vi "log analysis_gps.vi"() -> ()   [LabVIEW 2018] (continued)
2 28.000000 0 0\trobot status\t224.451032\t106.284325\t8.226800\t-0.416933\t-0.582279\t162.075425\t0.000000\t0.000000\n\t\n15:38:05.2\tlog_raw\tgps_raw\t\tsystem status\tnormal 2 28.000000 0 0\trobot status\t224.451188\t106.284516\t8.226800\t-0.415432\t-0.584104\t162.073380\t0.000000\t0.000000\n\t\n15:38:05.7\tlog_raw\tgps_raw\t#INSPVAXA,USB3,0,48.5,FINESTEERING,2107,283103.750,02000000,471d,15824;INS_ALIGNMENT_COMPLETE,INS_RTKFIXED,37.37108788000,126.72336903510,8.2270,22.3000,0.0050,0.0045,0.0003,-0.414277574,-0.583463216,287.925982879,0.2110,0.1573,0.2695,0.0344,0.0343,0.0312,0.0795,0.0805,4.9172,0f000005,0*7ee9c1ee\n\tsystem status\tnormal 2 28.000000 0 0\trobot status\t224.451369\t106.285108\t8.227000\t-0.414278\t-0.583463\t162.074017\t0.000000\t0.000000\n\t\n15:38:06.2\tlog_raw\tgps_raw\t#INSPVAXA,USB3,0,49.0,FINESTEERING,2107,283104.250,02000000,471d,15824;INS_ALIGNMENT_COMPLETE,INS_RTKFIXED,37.37108788419,126.72336903801,8.2270,22.3000,0.0052,0.0047,-0.0002,-0.414476277,-0.584193509,287.926239450,0.2108,0.1573,0.2688,0.0344,0.0343,0.0312,0.0795,0.0805,4.9186,0f000005,0*7089b505\n\tsystem status\tnormal 2 28.000000 0 0\trobot status\t224.451627\t106.285573\t8.227000\t-0.414476\t-0.584194\t162.073761\t0.000000\t0.000000\n\t\n15:38:06.7\tlog_raw\tgps_raw\t#INSPVAXA,USB3,0,49.0,FINESTEERING,2107,283104.750,02000000,471d,15824;INS_ALIGNMENT_COMPLETE,INS_RTKFIXED,37.37108788145,126.72336903923,8.2266,22.3000,0.0045,0.0040,-0.0007,-0.415917885,-0.588202727,287.926434552,0.2108,0.1573,0.2688,0.0344,0.0343,0.0312,0.0795,0.0805,4.9186,0f000005,0*a8fd5de4\n\tsystem status\tnormal 2 28.000000 0 0\trobot status\t224.451735\t106.285269\t8.226600\t-0.415918\t-0.588203\t162.073565\t0.000000\t0.000000\n\t\n15:38:07.2\tlog_raw\tgps_raw\t#INSPVAXA,USB3,0,48.0,FINESTEERING,2107,283105.250,02000000,471d,15824;INS_ALIGNMENT_COMPLETE,INS_RTKFIXED,37.37108788026,126.72336903795,8.2263,22.3000,0.0046,0.0032,-0.0010,-0.414361935,-0.591993164,287.925953212,0.2107,0.1573,0.2682,0.0344,0.0343,0.0312,0.0795,0.0805,4.9201,0f000005,0*118aea77\n\tsystem status\tnormal 2 28.000000 0 0\trobot status\t224.451622\t106.285136\t8.226300\t-0.414362\t-0.591993\t162.074047\t0.000000\t0.000000\n\t\n15:38:07.7\tlog_raw\tgps_raw\t#INSPVAXA,USB3,0,48.0,FINESTEERING,2107,283105.750,02000000,471d,15824;INS_ALIGNMENT_COMPLETE,INS_RTKFIXED,37.37108788332,126.72336903309,8.2260,22.3000,0.0050,0.0029,-0.0017,-0.412327684,-0.591969420,287.923357283,0.2107,0.1573,0.2682,0.0344,0.0343,0.0312,0.0795,0.0805,4.9201,0f000005,0*6e4f183a\n\tsystem status\tnormal 2 28.000000 0 0\trobot status\t224.451191\t106.285476\t8.226000\t-0.412328\t-0.591969\t162.076643\t0.000000\t0.000000\n\t\n15:38:08.2\tlog_raw\tgps_raw\t#INSPVAXA,USB3,0,48.5,FINESTEERING,2107,283106.250,02000000,471d,15824;INS_ALIGNMENT_COMPLETE,INS_RTKFIXED,37.37108788583,126.72336903030,8.2257,22.3000,0.0061,0.0025,-0.0021,-0.413322314,-0.593362730,287.923193741,0.2106,0.1573,0.2676,0.0344,0.0343,0.0312,0.0795,0.0805,4.9216,0f000005,0*8b1995f2\n\tsystem status\tnormal 2 28.000000 0 0\trobot status\t224.450944\t106.285755\t8.225700\t-0.413322\t-0.593363\t162.076806\t0.000000\t0.000000\n\t\n15:38:08.7\tlog_raw\tgps_raw\t#INSPVAXA,USB3,0,48.5,FINESTEERING,2107,283106.750,02000000,471d,15824;INS_ALIGNMENT_COMPLETE,INS_RTKFIXED,37.37108788780,126.72336903040,8.2256,22.3000,0.0063,0.0024,-0.0014,-0.411919741,-0.593309816,287.922053260,0.2106,0.1573,0.2676,0.0344,0.0343,0.0312,0.0795,0.0805,4.9216,0f000005,0*86796b00\n\tsystem status\tnormal 2 28.000000 0 0\trobot status\t224.450953\t106.285973\t8.225600\t-0.411920\t-0.593310\t162.077947\t0.000000\t0.000000\n\t\n15:38:09.2\tlog_raw\tgps_raw\t\tsystem status\tnormal 2 28.000000 0 0\trobot status\t224.450894\t106.286027\t8.225400\t-0.411158\t-0.594185\t162.080368\t0.000000\t0.000000\n\t\n15:38:09.7\tlog_raw\tgps_raw\t\tsystem status\tnormal 2 28.000000 0 0\trobot status\t224.450634\t106.285755\t8.225200\t-0.409687\t-0.594930\t162.079773\t0.000000\t0.000000\n\t\n15:38:10.2\tlog_raw\tgps_raw\t#INSPVAXA,USB3,0,49.0,FINESTEERING,2107,283108.250,02000000,471d,15824;INS_ALIGNMENT_COMPLETE,INS_RTKFIXED,37.37108788248,126.72336902361,8.2250,22.3000,0.0042,0.0015,-0.0018,-0.409863659,-0.598671820,287.918736221,0.2106,0.1573,0.2666,0.0344,0.0343,0.0312,0.0795,0.0805,4.9245,0f000005,0*9ed896c6\n\tsystem status\tnormal 2 28.000000 0 0\trobot status\t224.450352\t106.285383\t8.225000\t-0.409864\t-0.598672\t162.081264\t0.000000\t0.000000\n\t\n15:38:10.7\tlog_raw\tgps_raw\t#INSPVAXA,USB3,0,49.0,FINESTEERING,2107,283108.750,02000000,471d,15824;INS_ALIGNMENT_COMPLETE,INS_RTKFIXED,37.37108788055,126.72336902250,8.2249,22.3000,0.0042,0.0020,-0.0022,-0.409039214,-0.598045025,287.918760673,0.2106,0.1573,0.2666,0.0344,0.0343,0.0312,0.0795,0.0805,4.9245,0f000005,0*7d4209e8\n\tsystem status\tnormal 2 28.000000 0 0\trobot status\t224.450253\t106.285169\t8.224900\t-0.409039\t-0.598045\t162.081239\t0.000000\t0.000000\n\t\n15:38:11.2\tlog_raw\tgps_raw\t#INSPVAXA,USB3,0,49.0,FINESTEERING,2107,283109.250,02000000,471d,15824;INS_ALIGNMENT_COMPLETE,INS_RTKFIXED,37.37108788018,126.72336902226,8.2247,22.3000,0.0041,0.0020,-0.0021,-0.409961189,-0.600264889,287.916717631,0.2105,0.1573,0.2661,0.0344,0.0343,0.0312,0.0795,0.0805,4.9260,0f000005,0*bcf00a2d\n\tsystem status\tnormal 2 28.000000 0 0\trobot status\t224.450232\t106.285128\t8.224700\t-0.409961\t-0.600265\t162.083282\t0.000000\t0.000000\n\t\n15:38:11.7\tlog_raw\tgps_raw\t#INSPVAXA,USB3,0,49.0,FINESTEERING,2107,283109.750,02000000,471d,15824;INS_ALIGNMENT_COMPLETE,INS_RTKFIXED,37.37108788128,126.72336902017,8.2243,22.3000,0.0038,0.0017,-0.0025,-0.411876741,-0.602713375,287.916096171,0.2105,0.1573,0.2661,0.0344,0.0343,0.0312,0.0795,0.0805,4.9260,0f000005,0*0e51d129\n\tsystem status\tnormal 2 28.000000 0 0\trobot status\t224.450047\t106.285250\t8.224300\t-0.411877\t-0.602713\t162.083904\t0.000000\t0.000000\n\t\n15:38:12.2\tlog_raw\tgps_raw\t#INSPVAXA,USB3,0,47.0,FINESTEERING,2107,283110.250,02000000,471d,15824;INS_ALIGNMENT_COMPLETE,INS_RTKFIXED,37.37108788100,126.72336901819,8.2239,22.3000,0.0037,0.0018,-0.0030,-0.411621660,-0.604000034,287.914564647,0.2104,0.1573,0.2657,0.0344,0.0343,0.0312,0.0795,0.0805,4.9275,0f000005,0*d6cead36\n\tsystem status\tnormal 2 28.000000 0 0\trobot status\t224.449871\t106.285219\t8.223900\t-0.411622\t-0.604000\t162.085435\t0.000000\t0.000000\n\t\n15:38:12.7\tlog_raw\tgps_raw\t#INSPVAXA,USB3,0,47.0,FINESTEERING,2107,283110.750,02000000,471d,15824;INS_ALIGNMENT_COMPLETE,INS_RTKFIXED,37.37108787882,126.72336901490,8.2238,22.3000,0.0031,0.0013,-0.0034,-0.411270923,-0.605029312,287.914838543,0.2104,0.1573,0.2657,0.0344,0.0343,0.0312,0.0795,0.0805,4.9275,0f000005,0*6d07f4f4\n\tsystem status\tnormal 2 28.000000 0 0\trobot status\t224.449580\t106.284977\t8.223800\t-0.411271\t-0.605029\t162.085161\t0.000000\t0.000000\n\t\n15:38:13.2\tlog_raw\tgps_raw\t#INSPVAXA,USB3,0,44.0,FINESTEERING,2107,283111.250,02000000,471d,15824;INS_ALIGNMENT_COMPLETE,INS_RTKFIXED,37.37108787798,126.72336901339,8.2237,22.3000,0.0035,0.0008,-0.0027,-0.411014484,-0.606801614,287.916144015,0.2104,0.1572,0.2653,0.0344,0.0343,0.0312,0.0795,0.0805,4.9290,0f000005,0*17fda63e\n\tsystem status\tnormal 2 28.000000 0 0\trobot status\t224.449446\t106.284883\t8.223700\t-0.411014\t-0.606802\t162.083856\t0.000000\t0.000000\n\t\n15:38:13.7\tlog_raw\tgps_raw\t\tsystem status\tnormal 2 28.000000 0 0\trobot status\t224.449134\t106.285474\t8.223900\t-0.409737\t-0.609292\t162.084146\t0.000000\t0.000000\n\t\n15:38:14.2\tlog_raw\tgps_raw\t#INSPVAXA,USB3,0,46.5,FINESTEERING,2107,283112.250,02000000,471d,15824;INS_ALIGNMENT_COMPLETE,INS_RTKFIXED,37.37108788668,126.72336900523,8.2241,22.3000,0.0049,-0.0005,-0.0016,-0.408777501,-0.612185293,287.914677114,0.2103,0.1572,0.2649,0.0344,0.0343,0.0312,0.0795,0.0805,4.9305,0f000005,0*82ade194\n\tsystem status\tnormal 2 28.000000 0 0\trobot status\t224.448723\t106.285849\t8.224100\t-0.408778\t-0.612185\t162.085323\t0.000000\t0.000000\n\t\n15:38:14.7\tlog_raw\tgps_raw\t#INSPVAXA,USB3,0,46.5,FINESTEERING,2107,283112.750,02000000,471d,15824;INS_ALIGNMENT_COMPLETE,INS_RTKFIXED,37.37108788778,126.72336899951,8.2242,22.3000,0.0047,-0.0009,-0.0019,-0.409122282,-0.611972311,287.914890224,0.2103,0.1572,0.2649,0.0344,0.0343,0.0312,0.0795,0.0805,4.9305,0f000005,0*c3a4b162\n\tsystem status\tnormal 2 28.000000 0 0\trobot status\t224.448217\t106.285971\t8.224200\t-0.409122\t-0.611972\t162.085110\t0.000000\t0.000000\n\t\n15:38:15.2\tlog_raw\tgps_raw\t#INSPVAXA,USB3,0,48.5,FINESTEERING,2107,283113.250,02000000,471d,15824;INS_ALIGNMENT_COMPLETE,INS_RTKFIXED,37.37108788861,126.72336899425,8.2243,22.3000,0.0050,-0.0013,-0.0019,-0.410508140,-0.611024198,287.914176571,0.2103,0.1572,0.2646,0.0344,0.0343,0.0312,0.0795,0.0805,4.9321,0f000005,0*87d2d5b6\n\tsystem status\tnormal 2 28.000000 0 0\trobot status\t224.447751\t106.286063\t8.224300\t-0.410508\t-0.611024\t162.085823\t0.000000\t0.000000\n\t\n15:38:15.7\tlog_raw\tgps_raw\t#INSPVAXA,USB3,0,48.5,FINESTEERING,2107,283113.750,02000000,471d,15824;INS_ALIGNMENT_COMPLETE,INS_RTKFIXED,37.37108789363,126.72336898840,8.2244,22.3000,0.0063,-0.0021,-0.0017,-0.411022705,-0.609051513,287.913579305,0.2103,0.1572,0.2646,0.0344,0.0343,0.0312,0.0795,0.0805,4.9321,0f000005,0*35e79e67\n\tsystem status\tnormal 2 28.000000 0 0\trobot status\t224.447233\t106.286620\t8.224400\t-0.411023\t-0.609052\t162.086421\t0.000000\t0.000000\n\t\n15:38:16.2\tlog_raw\tgps_raw\t#INSPVAXA,USB3,0,47.0,FINESTEERING,2107,283114.250,02000000,471d,15824;INS_ALIGNMENT_COMPLETE,INS_RTKFIXED,37.37108789523,126.72336898295,8.2245,22.3000,0.0061,-0.0024,-0.0023,-0.410389175,-0.608679796,287.908436695,0.2102,0.1572,0.2643,0.0344,0.0343,0.0312,0.0795,0.0805,4.9336,0f000005,0*e900128e\n\tsystem status\tnormal 2 28.000000 0 0\trobot status\t224.446750\t106.286798\t8.224500\t-0.410389\t-0.608680\t162.091563\t0.000000\t0.000000\n\t\n15:38:16.7\tlog_raw\tgps_raw\t#INSPVAXA,USB3,0,47.0,FINESTEERING,2107,283114.750,02000000,471d,15824;INS_ALIGNMENT_COMPLETE,INS_RTKFIXED,37.37108789043,126.72336897889,8.2245,22.3000,0.0054,-0.0027,-0.0027,-0.410079836,-0.608000188,287.907030910,0.2102,0.1572,0.2643,0.0344,0.0343,0.0312,0.0795,0.0805,4.9336,0f000005,0*f5aa2bf4\n\tsystem status\tnormal 2 28.000000 0 0\trobot status\t224.446390\t106.286265\t8.224500\t-0.410080\t-0.608000\t162.092969\t0.000000\t0.000000\n\t\n15:38:17.2\tlog_raw\tgps_raw\t#INSPVAXA,USB3,0,46.0,FINESTEERING,2107,283115.250,02000000,471d,15824;INS_ALIGNMENT_COMPLETE,INS_RTKFIXED,37.37108788786,126.72336897498,8.2245,22.3000,0.0055,-0.0029,-0.0021,-0.409736809,-0.602715261,287.905938302,0.2101,0.1572,0.2640,0.0344,0.0343,0.0312,0.0795,0.0805,4.9352,0f000005,0*b8856e6c\n\tsystem status\tnormal 2 28.000000 0 0\trobot status\t224.446044\t106.285980\t8.224500\t-0.409737\t-0.602715\t162.094062\t0.000000\t0.000000\n\t\n15:38:17.7\tlog_raw\tgps_raw\t#INSPVAXA,USB3,0,46.0,FINESTEERING,2107,283115.750,02000000,471d,15824;INS_ALIGNMENT_COMPLETE,INS_RTKFIXED,37.37108788493,126.72336897577,8.2245,22.3000,0.0046,-0.0023,-0.0026,-0.410098984,-0.602405796,287.902959038,0.2101,0.1572,0.2640,0.0344,0.0343,0.0312,0.0795,0.0805,4.9352,0f000005,0*5724c76a\n\tsystem status\tnormal 2 28.000000 0 0\trobot status\t224.446114\t106.285655\t8.224500\t-0.410099\t-0.602406\t162.097041\t0.000000\t0.000000\n\t\n15:38:18.2\tlog_raw\tgps_raw\t\tsystem status\tnormal 2 28.000000 0 0\trobot status\t224.446206\t106.285296\t8.224400\t-0.410302\t-0.600878\t162.097351\t0.000000\t0.000000\n\t\n15:38:18.7\tlog_raw\tgps_raw\t\tsystem status\tnormal 2 28.000000 0 0\trobot status\t224.446412\t106.285047\t8.224500\t-0.408719\t-0.597692\t162.099652\t0.000000\t0.000000\n\t\n15:38:19.2\tlog_raw\tgps_raw\t#INSPVAXA,USB3,0,48.5,FINESTEERING,2107,283117.250,02000000,471d,15824;INS_ALIGNMENT_COMPLETE,INS_RTKFIXED,37.37108787822,126.72336898248,8.2247,22.3000,0.0046,0.0006,-0.0022,-0.408932053,-0.597708499,287.898385765,0.2100,0.1572,0.2634,0.0344,0.0343,0.0312,0.0795,0.0805,4.9381,0f000005,0*450763d8\n\tsystem status\tnormal 2 28.000000 0 0\trobot status\t224.446708\t106.284910\t8.224700\t-0.408932\t-0.597708\t162.101614\t0.000000\t0.000000\n\t\n15:38:19.7\tlog_raw\tgps_raw\t\tsystem status\tnormal 2 28.000000 0 0\trobot status\t224.446942\t106.284576\t8.225000\t-0.409149\t-0.598860\t162.102968\t0.000000\t0.000000\n\t\n15:38:20.2\tlog_raw\tgps_raw\t\tsystem status\tnormal 2 28.000000 0 0\trobot status\t224.447153\t106.284340\t8.225300\t-0.409921\t-0.598794\t162.103793\t0.000000\t0.000000\n\t\n15:38:20.7\tlog_raw\tgps_raw\t#INSPVAXA,USB3,0,51.5,FINESTEERING,2107,283118.750,02000000,471d,15824;INS_ALIGNMENT_COMPLETE,INS_RTKFIXED,37.37108787489,126.72336898888,8.2255,22.3000,0.0051,0.0006,-0.0004,-0.410553255,-0.597325999,287.895855349,0.2099,0.1572,0.2632,0.0344,0.0343,0.0312,0.0794,0.0805,4.9396,0f000005,0*531bbf8e\n\tsystem status\tnormal 2 28.000000 0 0\trobot status\t224.447275\t106.284541\t8.225500\t-0.410553\t-0.597326\t162.104145\t0.000000\t0.000000\n\t\n15:38:21.2\tlog_raw\tgps_raw\t\tsystem status\tnormal 2 28.000000 0 0\trobot status\t224.447208\t106.284839\t8.225600\t-0.411045\t-0.597182\t162.104666\t0.000000\t0.000000\n\t\n15:38:21.7\tlog_raw\tgps_raw\t#INSPVAXA,USB3,0,49.0,FINESTEERING,2107,283119.750,02000000,471d,15824;INS_ALIGNMENT_COMPLETE,INS_RTKFIXED,37.37108788239,126.72336898736,8.2256,22.3000,0.0062,0.0005,-0.0005,-0.410245690,-0.596223685,287.896349306,0.2099,0.1572,0.2630,0.0344,0.0343,0.0312,0.0794,0.0805,4.9410,0f000005,0*aabca186\n\tsystem status\tnormal 2 28.000000 0 0\trobot status\t224.447141\t106.285373\t8.225600\t-0.410246\t-0.596224\t162.103651\t0.000000\t0.000000\n\t\n15:38:22.2\tlog_raw\tgps_raw\t#INSPVAXA,USB3,0,47.5,FINESTEERING,2107,283120.250,02000000,471d,15824;INS_ALIGNMENT_COMPLETE,INS_RTKFIXED,37.37108788462,126.72336898711,8.2255,22.3000,0.0062,0.0002,-0.0014,-0.410019875,-0.596819628,287.894466218,0.2099,0.1572,0.2628,0.0344,0.0343,0.0312,0.0794,0.0805,4.9425,0f000005,0*feb71611\n\tsystem status\tnormal 2 28.000000 0 0\trobot status\t224.447118\t106.285620\t8.225500\t-0.410020\t-0.596820\t162.105534\t0.000000\t0.000000\n\t\n15:38:22.7\tlog_raw\tgps_raw\t\tsystem status\tnormal 2 28.000000 0 0\trobot status\t224.447175\t106.285403\t8.225200\t-0.411640\t-0.595952\t162.105189\t0.000000\t0.000000\n\t\n15:38:23.2\tlog_raw\tgps_raw\t#INSPVAXA,USB3,0,47.5,FINESTEERING,2107,283121.250,02000000,471d,15824;INS_ALIGNMENT_COMPLETE,INS_RTKFIXED,37.37108788020,126.72336899019,8.2251,22.3000,0.0049,0.0012,-0.0017,-0.410504520,-0.596359600,287.895045223,0.2098,0.1572,0.2627,0.0344,0.0343,0.0312,0.0794,0.0805,4.9439,0f000005,0*861abdab\n\tsystem status\tnormal 2 28.000000 0 0\trobot status\t224.447391\t106.285130\t8.225100\t-0.410505\t-0.596360\t162.104955\t0.000000\t0.000000\n\t\n15:38:23.7\tlog_raw\tgps_raw\t\tsystem status\tnormal 2 28.000000 0 0\trobot status\t224.447275\t106.285221\t8.225400\t-0.410985\t-0.596680\t162.105710\t0.000000\t0.000000\n\t\n15:38:24.2\tlog_raw\tgps_raw\t#INSPVAXA,USB3,0,48.0,FINESTEERING,2107,283122.250,02000000,471d,15824;INS_ALIGNMENT_COMPLETE,INS_RTKFIXED,37.37108788140,126.72336898679,8.2256,22.3000,0.0046,0.0003,-0.0020,-0.412214067,-0.597500472,287.894257245,0.2098,0.1572,0.2625,0.0344,0.0343,0.0312,0.0794,0.0805,4.9454,0f000005,0*41de74d7\n\tsystem status\tnormal 2 28.000000 0 0\trobot status\t224.447090\t106.285263\t8.225600\t-0.412214\t-0.597500\t162.105743\t0.000000\t0.000000\n\t\n15:38:24.7\tlog_raw\tgps_raw\t\tsystem status\tnormal 2 28.000000 0 0\trobot status\t224.447403\t106.284767\t8.225500\t-0.410260\t-0.595330\t162.106312\t0.000000\t0.000000\n\t\n15:38:25.2\tlog_raw\tgps_raw\t\tsystem status\tnormal 2 28.000000 0 0\trobot status\t224.447705\t106.284349\t8.225700\t-0.410048\t-0.596707\t162.108461\t0.000000\t0.000000\n\t\n15:38:25.7\tlog_raw\tgps_raw\t\tsystem status\tnormal 2 28.000000 0 0\trobot status\t224.447585\t106.284234\t8.226100\t-0.411201\t-0.596838\t162.109642\t0.000000\t0.000000\n\t\n15:38:26.2\tlog_raw\tgps_raw\t\tsystem status\tnormal 2 28.000000 0 0\trobot status\t224.447570\t106.283848\t8.226500\t-0.410870\t-0.598506\t162.111627\t0.000000\t0.000000\n\t\n15:38:26.7\tlog_raw\tgps_raw\t\tsystem status\tnormal 2 28.000000 0 0\trobot status\t224.447639\t106.283383\t8.226500\t-0.408777\t-0.600718\t162.112837\t0.000000\t0.000000\n\t\n15:38:27.2\tlog_raw\tgps_raw\t\tsystem status\tnormal 2 28.000000 0 0\trobot status\t224.447605\t106.283011\t8.226500\t-0.406755\t-0.601265\t162.115733\t0.000000\t0.000000\n\t\n15:38:27.7\tlog_raw\tgps_raw\t\tsystem status\tnormal 2 28.000000 0 0\trobot status\t224.447669\t106.282715\t8.226400\t-0.405589\t-0.600901\t162.115380\t0.000000\t0.000000\n\t\n15:38:28.2\tlog_raw\tgps_raw\t#INSPVAXA,USB3,0,46.5,FINESTEERING,2107,283126.250,02000000,471d,15824;INS_ALIGNMENT_COMPLETE,INS_RTKFIXED,37.37108785781,126.72336899407,8.2263,22.3000,0.0034,0.0010,-0.0014,-0.405163325,-0.599911050,287.885200973,0.2098,0.1572,0.2620,0.0344,0.0343,0.0312,0.0794,0.0804,4.9511,0f000005,0*554930fc\n\tsystem status\tnormal 2 28.000000 0 0\trobot status\t224.447735\t106.282645\t8.226300\t-0.405163\t-0.599911\t162.114799\t0.000000\t0.000000\n\t\n15:38:28.7\tlog_raw\tgps_raw\t\tsystem status\tnormal 2 28.000000 0 0\trobot status\t224.447887\t106.282579\t8.226100\t-0.406198\t-0.601239\t162.115348\t0.000000\t0.000000\n\t\n15:38:29.2\tlog_raw\tgps_raw\t\tsystem status\tnormal 2 28.000000 0 0\trobot status\t224.447997\t106.282609\t8.225900\t-0.407404\t-0.600387\t162.116168\t0.000000\t0.000000\n\t\n15:38:29.7\tlog_raw\tgps_raw\t\tsystem status\tnormal 2 28.000000 0 0\trobot status\t224.448154\t106.282775\t8.225900\t-0.406329\t-0.599457\t162.114574\t0.000000\t0.000000\n\t\n15:38:30.2\tlog_raw\tgps_raw\t\tsystem status\tnormal 2 28.000000 0 0\trobot status\t224.448312\t106.282869\t8.225900\t-0.405480\t-0.599703\t162.115826\t0.000000\t0.000000\n\t\n15:38:30.7\tlog_raw\tgps_raw\t\tsystem status\tnormal 2 28.000000 0 0\trobot status\t224.448419\t106.282962\t8.225800\t-0.403880\t-0.599318\t162.116186\t0.000000\t0.000000\n\t\n15:38:31.2\tlog_raw\tgps_raw\t\tsystem status\tnormal 2 28.000000 0 0\trobot status\t224.448426\t106.283107\t8.225500\t-0.401514\t-0.597654\t162.115583\t0.000000\t0.000000\n\t\n15:38:31.7\tlog_raw\tgps_raw\t\tsystem status\tnormal 2 28.000000 0 0\trobot status\t224.448410\t106.283254\t8.225400\t-0.401145\t-0.595126\t162.115399\t0.000000\t0.000000\n\t\n15:38:32.2\tlog_raw\tgps_raw\t\tsystem status\tnormal 2 28.000000 0 0\trobot status\t224.448462\t106.283450\t8.225300\t-0.398774\t-0.594293\t162.114275\t0.000000\t0.000000\n\t\n15:38:32.7\tlog_raw\tgps_raw\t\tsystem status\tnormal 2 28.000000 0 0\trobot status\t224.448562\t106.283708\t8.225500\t-0.399325\t-0.595095\t162.114742\t0.000000\t0.000000\n\t\n15:38:33.2\tlog_raw\tgps_raw\t\tsystem status\tnormal 2 28.000000 0 0\trobot status\t224.448698\t106.283907\t8.225600\t-0.399060\t-0.595550\t162.114322\t0.000000\t0.000000\n\t\n15:38:33.7\tlog_raw\tgps_raw\t\tsystem status\tnormal 2 28.000000 0 0\trobot status\t224.449149\t106.284287\t8.225700\t-0.398384\t-0.595717\t162.114541\t0.000000\t0.000000\n\t\n15:38:34.2\tlog_raw\tgps_raw\t\tsystem status\tnormal 2 28.000000 0 0\trobot status\t224.449553\t106.284564\t8.225700\t-0.399591\t-0.594833\t162.114493\t0.000000\t0.000000\n\t\n15:38:34.7\tlog_raw\tgps_raw\t\tsystem status\tnormal 2 28.000000 0 0\trobot status\t224.449775\t106.284492\t8.225300\t-0.400663\t-0.594497\t162.113796\t0.000000\t0.000000\n\t\n15:38:35.2\tlog_raw\tgps_raw\t#INSPVAXA,USB3,0,50.5,FINESTEERING,2107,283133.250,02008000,471d,15824;INS_ALIGNMENT_COMPLETE,INS_RTKFIXED,37.37108787441,126.72336901696,8.2251,22.3000,0.0051,0.0025,0.0013,-0.401038405,-0.592309574,287.886306258,0.2098,0.1572,0.2615,0.0344,0.0343,0.0312,0.0794,0.0804,4.9611,0f000005,0*3f736d45\n\tsystem status\tnormal 2 28.000000 0 0\trobot status\t224.449763\t106.284487\t8.225100\t-0.401038\t-0.592310\t162.113694\t0.000000\t0.000000\n\t\n15:38:35.7\tlog_raw\tgps_raw\t\tsystem status\tnormal 2 28.000000 0 0\trobot status\t224.449857\t106.284844\t8.225400\t-0.401355\t-0.592289\t162.114419\t0.000000\t0.000000\n\t\n15:38:36.2\tlog_raw\tgps_raw\t\tsystem status\tnormal 2 28.000000 0 0\trobot status\t224.450031\t106.285085\t8.225500\t-0.401303\t-0.591132\t162.115391\t0.000000\t0.000000\n\t\n15:38:36.7\tlog_raw\tgps_raw\t\tsystem status\tnormal 2 28.000000 0 0\trobot status\t224.450093\t106.285122\t8.225700\t-0.403482\t-0.591750\t162.114729\t0.000000\t0.000000\n\t\n15:38:37.2\tlog_raw\tgps_raw\t\tsystem status\tnormal 2 28.000000 0 0\trobot status\t224.450414\t106.285141\t8.225700\t-0.404978\t-0.591486\t162.114393\t0.000000\t0.000000\n\t\n15:38:37.7\tlog_raw\tgps_raw\t\tsystem status\tnormal 2 28.000000 0 0\trobot status\t224.451129\t106.285112\t8.225400\t-0.405382\t-0.592732\t162.113860\t0.000000\t0.000000\n\t\n15:38:38.2\tlog_raw\tgps_raw\t\tsystem status\tnormal 2 28.000000 0 0\trobot status\t224.451492\t106.285138\t8.225200\t-0.406408\t-0.593386\t162.114550\t0.000000\t0.000000\n\t\n15:38:38.7\tlog_raw\tgps_raw\t\tsystem status\tnormal 2 28.000000 0 0\trobot status\t224.451405\t106.285118\t8.224900\t-0.407947\t-0.592162\t162.114919\t0.000000\t0.000000\n\t\n15:38:39.2\tlog_raw\tgps_raw\t\tsystem status\tnormal 2 28.000000 0 0\trobot status\t224.451215\t106.285206\t8.224600\t-0.409714\t-0.592940\t162.113033\t0.000000\t0.000000\n\t\n15:38:39.7\tlog_raw\tgps_raw\t\tsystem status\tnormal 2 28.000000 0 0\trobot status\t224.451197\t106.285185\t8.224200\t-0.410417\t-0.593710\t162.112017\t0.000000\t0.000000\n\t\n15:38:40.2\tlog_raw\tgps_raw\t\tsystem status\tnormal 2 28.000000 0 0\trobot status\t224.451087\t106.285125\t8.223800\t-0.410324\t-0.597206\t162.111988\t0.000000\t0.000000\n\t\n15:38:40.7\tlog_raw\tgps_raw\t\tsystem status\tnormal 2 28.000000 0 0\trobot status\t224.450903\t106.285100\t8.223300\t-0.410450\t-0.598032\t162.111967\t0.000000\t0.000000\n\t\n15:38:41.3\tlog_raw\tgps_raw\t\tsystem status\tnormal 2 28.000000 0 0\trobot status\t224.450585\t106.285039\t8.222700\t-0.408179\t-0.598817\t162.113262\t0.000000\t0.000000\n\t\n15:38:41.8\tlog_raw\tgps_raw\t\tsystem status\tnormal 2 28.000000 0 0\trobot status\t224.449934\t106.285203\t8.222300\t-0.409129\t-0.601002\t162.114314\t0.000000\t0.000000\n\t\n15:38:42.3\tlog_raw\tgps_raw\t\tsystem status\tnormal 2 28.000000 0 0\trobot status\t224.449799\t106.285271\t8.222000\t-0.410425\t-0.600335\t162.112811\t0.000000\t0.000000\n\t\n15:38:42.8\tlog_raw\tgps_raw\t\tsystem status\tnormal 2 28.000000 0 0\trobot status\t224.450317\t106.284770\t8.221800\t-0.411049\t-0.600342\t162.114798\t0.000000\t0.000000\n\t\n15:38:43.3\tlog_raw\tgps_raw\t\tsystem status\tnormal 2 28.000000 0 0\trobot status\t224.450564\t106.284254\t8.221600\t-0.410176\t-0.599924\t162.113590\t0.000000\t0.000000\n\t\n15:38:43.8\tlog_raw\tgps_raw\t\tsystem status\tnormal 2 28.000000 0 0\trobot status\t224.450436\t106.283367\t8.221300\t-0.411311\t-0.599715\t162.114209\t0.000000\t0.000000\n\t\n15:38:44.3\tlog_raw\tgps_raw\t\tsystem status\tnormal 2 28.000000 0 0\trobot status\t224.450212\t106.282766\t8.221200\t-0.411664\t-0.598224\t162.112656\t0.000000\t0.000000\n\t\n15:38:44.8\tlog_raw\tgps_raw\t\tsystem status\tnormal 2 28.000000 0 0\trobot status\t224.449709\t106.282748\t8.221300\t-0.409737\t-0.601474\t162.113670\t0.000000\t0.000000\n\t\n15:38:45.3\tlog_raw\tgps_raw\t\tsystem status\tnormal 2 28.000000 0 0\trobot status\t224.449349\t106.282704\t8.221400\t-0.409268\t-0.601896\t162.113492\t0.000000\t0.000000\n\t\n15:38:45.8\tlog_raw\tgps_raw\t\tsystem status\tnormal 2 28.000000 0 0\trobot status\t224.449502\t106.282633\t8.221400\t-0.409607\t-0.601683\t162.113014\t0.000000\t0.000000\n\t\n15:38:46.3\tlog_raw\tgps_raw\t\tsystem status\tnormal 2 28.000000 0 0\trobot status\t224.449611\t106.282613\t8.221300\t-0.408273\t-0.601250\t162.114429\t0.000000\t0.000000\n\t\n15:38:46.8\tlog_raw\tgps_raw\t\tsystem status\tnormal 2 28.000000 0 0\trobot status\t224.449703\t106.282874\t8.221200\t-0.406329\t-0.598269\t162.116793\t0.000000\t0.000000\n\t\n15:38:47.3\tlog_raw\tgps_raw\t\tsystem status\tnormal 2 28.000000 0 0\trobot status\t224.449773\t106.283158\t8.221000\t-0.408057\t-0.601140\t162.117271\t0.000000\t0.000000\n\t\n15:38:47.8\tlog_raw\tgps_raw\t#INSPVAXA,USB3,0,50.0,FINESTEERING,2107,283145.800,02000000,471d,15824;INS_ALIGNMENT_COMPLETE,INS_RTKFIXED,37.37108786440,126.72336901151,8.2210,22.3000,0.0034,-0.0002,0.0004,-0.408176107,-0.602369941,287.881922019,0.2098,0.1572,0.2612,0.0344,0.0343,0.0312,0.0794,0.0804,4.9785,0f000005,0*1b1c4bf8\n\tsystem status\tnormal 2 28.000000 0 0\trobot status\t224.449280\t106.283376\t8.221000\t-0.408176\t-0.602370\t162.118078\t0.000000\t0.000000\n\t\n15:38:48.3\tlog_raw\tgps_raw\t\tsystem status\tnormal 2 28.000000 0 0\trobot status\t224.448891\t106.283426\t8.221100\t-0.406468\t-0.603285\t162.120910\t0.000000\t0.000000\n\t\n15:38:48.8\tlog_raw\tgps_raw\t\tsystem status\tnormal 2 28.000000 0 0\trobot status\t224.448305\t106.283588\t8.221000\t-0.407126\t-0.603090\t162.122796\t0.000000\t0.000000\n\t\n15:38:49.3\tlog_raw\tgps_raw\t\tsystem status\tnormal 2 28.000000 0 0\trobot status\t224.447906\t106.283751\t8.221000\t-0.407221\t-0.604315\t162.125806\t0.000000\t0.000000\n\t\n15:38:49.8\tlog_raw\tgps_raw\t\tsystem status\tnormal 2 28.000000 0 0\trobot status\t224.448036\t106.283990\t8.221100\t-0.408565\t-0.603124\t162.125101\t0.000000\t0.000000\n\t\n15:38:50.3\tlog_raw\tgps_raw\t\tsystem status\tnormal 2 28.000000 0 0\trobot status\t224.448125\t106.284134\t8.221100\t-0.409333\t-0.603590\t162.125582\t0.000000\t0.000000\n\t\n15:38:50.8\tlog_raw\tgps_raw\t\tsystem status\tnormal 2 28.000000 0 0\trobot status\t224.447801\t106.284438\t8.221200\t-0.409831\t-0.602731\t162.126983\t0.000000\t0.000000\n\t\n15:38:51.3\tlog_raw\tgps_raw\t\tsystem status\tnormal 2 28.000000 0 0\trobot status\t224.447408\t106.284827\t8.221200\t-0.410804\t-0.599889\t162.128281\t0.000000\t0.000000\n\t\n15:38:51.8\tlog_raw\tgps_raw\t\tsystem status\tnormal 2 28.000000 0 0\trobot status\t224.447241\t106.284776\t8.221200\t-0.410682\t-0.600129\t162.129801\t0.000000\t0.000000\n\t\n15:38:52.3\tlog_raw\tgps_raw\t\tsystem status\tnormal 2 28.000000 0 0\trobot status\t224.447158\t106.284667\t8.221300\t-0.408685\t-0.599583\t162.132418\t0.000000\t0.000000\n\t\n15:38:52.8\tlog_raw\tgps_raw\t\tsystem status\tnormal 2 28.000000 0 0\trobot status\t224.447103\t106.284494\t8.221500\t-0.406064\t-0.598443\t162.134560\t0.000000\t0.000000\n\t\n15:38:53.3\tlog_raw\tgps_raw\t\tsystem status\tnormal 2 28.000000 0 0\trobot status\t224.447120\t106.284278\t8.221700\t-0.404946\t-0.597272\t162.134694\t0.000000\t0.000000\n\t\n15:38:53.8\tlog_raw\tgps_raw\t#INSPVAXA,USB3,0,45.5,FINESTEERING,2107,283151.800,02000000,471d,15824;INS_ALIGNMENT_COMPLETE,INS_RTKFIXED,37.37108787046,126.72336898866,8.2212,22.3000,0.0033,0.0009,-0.0006,-0.404916149,-0.597406910,287.865620586,0.2099,0.1572,0.2612,0.0344,0.0343,0.0312,0.0793,0.0804,4.9878,0f000005,0*a5f125e6\n\tsystem status\tnormal 2 28.000000 0 0\trobot status\t224.447256\t106.284049\t8.221200\t-0.404916\t-0.597407\t162.134379\t0.000000\t0.000000\n\t\n15:38:54.3\tlog_raw\tgps_raw\t#INSPVAXA,USB3,0,45.0,FINESTEERING,2107,283152.300,02000000,471d,15824;INS_ALIGNMENT_COMPLETE,INS_RTKFIXED,37.37108786806,126.72336899217,8.2208,22.3000,0.0029,0.0018,-0.0009,-0.404359469,-0.596798726,287.864856489,0.2099,0.1572,0.2612,0.0344,0.0343,0.0312,0.0793,0.0804,4.9892,0f000005,0*75438a82\n\tsystem status\tnormal 2 28.000000 0 0\trobot status\t224.447567\t106.283783\t8.220800\t-0.404359\t-0.596799\t162.135144\t0.000000\t0.000000\n\t\n15:38:54.8\tlog_raw\tgps_raw\t\tsystem status\tnormal 2 28.000000 0 0\trobot status\t224.447884\t106.283783\t8.220600\t-0.405343\t-0.597710\t162.135676\t0.000000\t0.000000\n\t\n15:38:55.3\tlog_raw\tgps_raw\t\tsystem status\tnormal 2 28.000000 0 0\trobot status\t224.448057\t106.283805\t8.220400\t-0.404579\t-0.599213\t162.136449\t0.000000\t0.000000\n\t\n15:38:55.8\tlog_raw\tgps_raw\t#INSPVAXA,USB3,0,47.5,FINESTEERING,2107,283153.800,02000000,471d,15824;INS_ALIGNMENT_COMPLETE,INS_RTKFIXED,37.37108786600,126.72336899902,8.2205,22.3000,0.0026,0.0021,-0.0023,-0.403425682,-0.598266477,287.862635982,0.2098,0.1572,0.2612,0.0344,0.0343,0.0312,0.0793,0.0804,4.9906,0f000005,0*5c2a9c66\n\tsystem status\tnormal 2 28.000000 0 0\trobot status\t224.448173\t106.283554\t8.220500\t-0.403426\t-0.598266\t162.137364\t0.000000\t0.000000\n\t\n15:38:56.3\tlog_raw\tgps_raw\t\tsystem status\tnormal 2 28.000000 0 0\trobot status\t224.448297\t106.283454\t8.220400\t-0.401893\t-0.599203\t162.136631\t0.000000\t0.000000\n\t\n15:38:56.8\tlog_raw\tgps_raw\t\tsystem status\tnormal 2 28.000000 0 0\trobot status\t224.448255\t106.283758\t8.220200\t-0.401745\t-0.600370\t162.138515\t0.000000\t0.000000\n\t\n15:38:57.3\tlog_raw\tgps_raw\t\tsystem status\tnormal 2 28.000000 0 0\trobot status\t224.448063\t106.283837\t8.220100\t-0.398830\t-0.598855\t162.138732\t0.000000\t0.000000\n\t\n15:38:57.8\tlog_raw\tgps_raw\t#INSPVAXA,USB3,0,49.0,FINESTEERING,2107,283155.800,02000000,471d,15824;INS_ALIGNMENT_COMPLETE,INS_RTKFIXED,37.37108786878,126.72336899361,8.2202,22.3000,0.0032,0.0004,-0.0022,-0.395795579,-0.599014783,287.862450492,0.2098,0.1572,0.2612,0.0344,0.0343,0.0312,0.0793,0.0804,4.9935,0f000005,0*f4cd5051\n\tsystem status\tnormal 2 28.000000 0 0\trobot status\t224.447694\t106.283862\t8.220200\t-0.395796\t-0.599015\t162.137550\t0.000000\t0.000000\n\t\n15:38:58.3\tlog_raw\tgps_raw\t#INSPVAXA,USB3,0,46.5,FINESTEERING,2107,283156.300,02000000,471d,15824;INS_ALIGNMENT_COMPLETE,INS_RTKFIXED,37.37108786919,126.72336899093,8.2205,22.3000,0.0038,-0.0001,-0.0013,-0.396437672,-0.598313647,287.862503112,0.2098,0.1572,0.2612,0.0344,0.0343,0.0312,0.0793,0.0804,4.9950,0f000005,0*5aa32664\n\tsystem status\tnormal 2 28.000000 0 0\trobot status\t224.447457\t106.283908\t8.220500\t-0.396438\t-0.598314\t162.137497\t0.000000\t0.000000\n\t\n15:38:58.8\tlog_raw\tgps_raw\t#INSPVAXA,USB3,0,46.5,FINESTEERING,2107,283156.800,02000000,471d,15824;INS_ALIGNMENT_COMPLETE,INS_RTKFIXED,37.37108787385,126.72336898941,8.2207,22.3000,0.0043,-0.0002,-0.0010,-0.392731293,-0.598638690,287.862042656,0.2098,0.1572,0.2612,0.0344,0.0343,0.0312,0.0793,0.0804,4.9950,0f000005,0*03d612e4\n\tsystem status\tnormal 2 28.000000 0 0\trobot status\t224.447322\t106.284425\t8.220700\t-0.392731\t-0.598639\t162.137957\t0.000000\t0.000000\n\t\n15:38:59.3\tlog_raw\tgps_raw\t#INSPVAXA,USB3,0,51.0,FINESTEERING,2107,283157.300,02000000,471d,15824;INS_ALIGNMENT_COMPLETE,INS_RTKFIXED,37.37108787685,126.72336898846,8.2211,22.3000,0.0052,-0.0002,-0.0000,-0.390778583,-0.597437105,287.863000385,0.2098,0.1573,0.2612,0.0344,0.0343,0.0312,0.0793,0.0804,4.9965,0f000005,0*3bc0d928\n\tsystem status\tnormal 2 28.000000 0 0\trobot status\t224.447238\t106.284758\t8.221100\t-0.390779\t-0.597437\t162.137000\t0.000000\t0.000000\n\t\n15:38:59.8\tlog_raw\tgps_raw\t\tsystem status\tnormal 2 28.000000 0 0\trobot status\t224.447056\t106.285291\t8.221800\t-0.390567\t-0.595531\t162.139186\t0.000000\t0.000000\n\t\n15:39:00.3\tlog_raw\tgps_raw\t\tsystem status\tnormal 2 28.000000 0 0\trobot status\t224.447010\t106.285438\t8.222200\t-0.388610\t-0.593673\t162.139248\t0.000000\t0.000000\n\t\n15:39:00.8\tlog_raw\tgps_raw\t\tsystem status\tnormal 2 28.000000 0 0\trobot status\t224.447483\t106.285521\t8.222200\t-0.387582\t-0.594521\t162.138949\t0.000000\t0.000000\n\t\n15:39:01.3\tlog_raw\tgps_raw\t#INSPVAXA,USB3,0,50.5,FINESTEERING,2107,283159.300,02000000,471d,15824;INS_ALIGNMENT_COMPLETE,INS_RTKFIXED,37.37108788569,126.72336899544,8.2223,22.3000,0.0068,0.0019,0.0013,-0.387086330,-0.593973069,287.861144002,0.2098,0.1573,0.2612,0.0344,0.0343,0.0312,0.0793,0.0803,4.9994,0f000005,0*0ed095af\n\tsystem status\tnormal 2 28.000000 0 0\trobot status\t224.447856\t106.285739\t8.222300\t-0.387086\t-0.593973\t162.138856\t0.000000\t0.000000\n\t\n15:39:01.8\tlog_raw\tgps_raw\t\tsystem status\tnormal 2 28.000000 0 0\trobot status\t224.447883\t106.286267\t8.222300\t-0.387070\t-0.594035\t162.138120\t0.000000\t0.000000\n\t\n15:39:02.3\tlog_raw\tgps_raw\t\tsystem status\tnormal 2 28.000000 0 0\trobot status\t224.448173\t106.286739\t8.222200\t-0.386894\t-0.594155\t162.137281\t0.000000\t0.000000\n\t\n15:39:02.8\tlog_raw\tgps_raw\t#INSPVAXA,USB3,0,44.5,FINESTEERING,2107,283160.800,02000000,471d,15824;INS_ALIGNMENT_COMPLETE,INS_RTKFIXED,37.37108790025,126.72336900642,8.2224,22.3000,0.0087,0.0034,0.0012,-0.385305357,-0.593887975,287.861236180,0.2098,0.1573,0.2612,0.0344,0.0343,0.0312,0.0793,0.0803,5.0008,0f000005,0*a535fac5\n\tsystem status\tnormal 2 28.000000 0 0\trobot status\t224.448829\t106.287355\t8.222400\t-0.385305\t-0.593888\t162.138764\t0.000000\t0.000000\n\t\n15:39:03.3\tlog_raw\tgps_raw\t\tsystem status\tnormal 2 28.000000 0 0\trobot status\t224.449174\t106.287808\t8.222400\t-0.384957\t-0.592216\t162.137898\t0.000000\t0.000000\n\t\n15:39:03.8\tlog_raw\tgps_raw\t#INSPVAXA,USB3,0,47.0,FINESTEERING,2107,283161.800,02000000,471d,15824;INS_ALIGNMENT_COMPLETE,INS_RTKFIXED,37.37108791058,126.72336901739,8.2224,22.3000,0.0091,0.0053,0.0008,-0.384677214,-0.593155644,287.863440186,0.2098,0.1573,0.2612,0.0344,0.0343,0.0312,0.0793,0.0803,5.0020,0f000005,0*15bd2f54\n\tsystem status\tnormal 2 28.000000 0 0\trobot status\t224.449801\t106.288502\t8.222400\t-0.384677\t-0.593156\t162.136560\t0.000000\t0.000000\n\t\n15:39:04.3\tlog_raw\tgps_raw\t#INSPVAXA,USB3,0,49.0,FINESTEERING,2107,283162.300,02000000,471d,15824;INS_ALIGNMENT_COMPLETE,INS_RTKFIXED,37.37108791275,126.72336902289,8.2223,22.3000,0.0092,0.0053,0.0006,-0.383976052,-0.593983766,287.863552246,0.2098,0.1573,0.2612,0.0344,0.0343,0.0312,0.0793,0.0803,5.0033,0f000005,0*f7f4aafb\n\tsystem status\tnormal 2 28.000000 0 0\trobot status\t224.450288\t106.288742\t8.222300\t-0.383976\t-0.593984\t162.136448\t0.000000\t0.000000\n\t\n15:39:04.8\tlog_raw\tgps_raw\t#INSPVAXA,USB3,0,49.0,FINESTEERING,2107,283162.800,02000000,471d,15824;INS_ALIGNMENT_COMPLETE,INS_RTKFIXED,37.37108791707,126.72336902756,8.2221,22.3000,0.0099,0.0052,0.0004,-0.383244439,-0.593582797,287.863703162,0.2098,0.1573,0.2612,0.0344,0.0343,0.0312,0.0793,0.0803,5.0033,0f000005,0*87119b1a\n\tsystem status\tnormal 2 28.000000 0 0\trobot status\t224.450701\t106.289222\t8.222100\t-0.383244\t-0.593583\t162.136297\t0.000000\t0.000000\n\t\n15:39:05.3\tlog_raw\tgps_raw\t#INSPVAXA,USB3,0,50.0,FINESTEERING,2107,283163.300,02000000,471d,15824;INS_ALIGNMENT_COMPLETE,INS_RTKFIXED,37.37108791768,126.72336903031,8.2218,22.3000,0.0093,0.0052,-0.0002,-0.382087992,-0.594481290,287.864257970,0.2098,0.1573,0.2612,0.0344,0.0343,0.0312,0.0793,0.0803,5.0046,0f000005,0*64efd3fe\n\tsystem status\tnormal 2 28.000000 0 0\trobot status\t224.450945\t106.289290\t8.221800\t-0.382088\t-0.594481\t162.135742\t0.000000\t0.000000\n\t\n15:39:05.8\tlog_raw\tgps_raw\t#INSPVAXA,USB3,0,50.0,FINESTEERING,2107,283163.800,02000000,471d,15824;INS_ALIGNMENT_COMPLETE,INS_RTKFIXED,37.37108791823,126.72336903544,8.2213,22.3000,0.0087,0.0054,-0.0002,-0.381855357,-0.594537838,287.865100598,0.2098,0.1573,0.2612,0.0344,0.0343,0.0312,0.0793,0.0803,5.0046,0f000005,0*eaa89ec3\n\tsystem status\tnormal 2 28.000000 0 0\trobot status\t224.451399\t106.289351\t8.221300\t-0.381855\t-0.594538\t162.134899\t0.000000\t0.000000\n\t\n15:39:06.3\tlog_raw\tgps_raw\t#INSPVAXA,USB3,0,49.5,FINESTEERING,2107,283164.300,02000000,471d,15824;INS_ALIGNMENT_COMPLETE,INS_RTKFIXED,37.37108791762,126.72336903818,8.2211,22.3000,0.0096,0.0053,-0.0000,-0.380427968,-0.595358698,287.865754120,0.2100,0.1573,0.2613,0.0344,0.0343,0.0312,0.0793,0.0803,5.0060,0f000005,0*9eb07253\n\tsystem status\tnormal 2 28.000000 0 0\trobot status\t224.451642\t106.289283\t8.221100\t-0.380428\t-0.595359\t162.134246\t0.000000\t0.000000\n\t\n15:39:06.8\tlog_raw\tgps_raw\t#INSPVAXA,USB3,0,49.5,FINESTEERING,2107,283164.800,02000000,471d,15824;INS_ALIGNMENT_COMPLETE,INS_RTKFIXED,37.37108792129,126.72336904200,8.2211,22.3000,0.0095,0.0050,0.0001,-0.381479450,-0.593246291,287.867192627,0.2100,0.1573,0.2613,0.0344,0.0343,0.0312,0.0793,0.0803,5.0060,0f000005,0*81097ed9\n\tsystem status\tnormal 2 28.000000 0 0\trobot status\t224.451981\t106.289690\t8.221100\t-0.381479\t-0.593246\t162.132807\t0.000000\t0.000000\n\t\n15:39:07.3\tlog_raw\tgps_raw\t#INSPVAXA,USB3,0,48.5,FINESTEERING,2107,283165.300,02000000,471d,15824;INS_ALIGNMENT_COMPLETE,INS_RTKFIXED,37.37108792359,126.72336904372,8.2212,22.3000,0.0098,0.0050,0.0003,-0.382461437,-0.592905475,287.870739528,0.2103,0.1573,0.2614,0.0344,0.0343,0.0312,0.0793,0.0803,5.0073,0f000005,0*f350cda0\n\tsystem status\tnormal 2 28.000000 0 0\trobot status\t224.452133\t106.289945\t8.221200\t-0.382461\t-0.592905\t162.129260\t0.000000\t0.000000\n\t\n15:39:07.8\tlog_raw\tgps_raw\t#INSPVAXA,USB3,0,48.5,FINESTEERING,2107,283165.800,02000000,471d,15824;INS_ALIGNMENT_COMPLETE,INS_RTKFIXED,37.37108792768,126.72336904655,8.2215,22.3000,0.0096,0.0053,0.0004,-0.381584283,-0.591456419,287.872579847,0.2103,0.1573,0.2614,0.0344,0.0343,0.0312,0.0793,0.0803,5.0073,0f000005,0*a9ef8806\n\tsystem status\tnormal 2 28.000000 0 0\trobot status\t224.452384\t106.290399\t8.221500\t-0.381584\t-0.591456\t162.127420\t0.000000\t0.000000\n\t\n15:39:08.3\tlog_raw\tgps_raw\t#INSPVAXA,USB3,0,47.0,FINESTEERING,2107,283166.300,02000000,471d,15824;INS_ALIGNMENT_COMPLETE,INS_RTKFIXED,37.37108793024,126.72336904905,8.2215,22.3000,0.0104,0.0057,0.0003,-0.382222726,-0.592164318,287.872646767,0.2105,0.1573,0.2615,0.0344,0.0343,0.0312,0.0793,0.0803,5.0087,0f000005,0*6f064ef0\n\tsystem status\tnormal 2 28.000000 0 0\trobot status\t224.452605\t106.290683\t8.221500\t-0.382223\t-0.592164\t162.127353\t0.000000\t0.000000\n\t\n15:39:08.8\tlog_raw\tgps_raw\t#INSPVAXA,USB3,0,47.0,FINESTEERING,2107,283166.800,02000000,471d,15824;INS_ALIGNMENT_COMPLETE,INS_RTKFIXED,37.37108793672,126.72336905212,8.2216,22.3000,0.0107,0.0058,0.0001,-0.380800259,-0.589429313,287.874913684,0.2105,0.1573,0.2615,0.0344,0.0343,0.0312,0.0793,0.0803,5.0087,0f000005,0*ee96ecc4\n\tsystem status\tnormal 2 28.000000 0 0\trobot status\t224.452877\t106.291403\t8.221600\t-0.380800\t-0.589429\t162.125086\t0.000000\t0.000000\n\t\n15:39:09.3\tlog_raw\tgps_raw\t#INSPVAXA,USB3,0,48.0,FINESTEERING,2107,283167.300,02000000,471d,15824;INS_ALIGNMENT_COMPLETE,INS_RTKFIXED,37.37108797180,126.72336907746,8.2214,22.3000,0.0123,0.0072,-0.0009,-0.380175638,-0.588519598,287.873648229,0.2105,0.1573,0.2615,0.0344,0.0343,0.0312,0.0793,0.0803,5.0087,0f000005,0*c5785aa0\n\tsystem status\tnormal 2 28.000000 0 0\trobot status\t224.455122\t106.295296\t8.221400\t-0.380176\t-0.588520\t162.126352\t0.000000\t0.000000\n\t\n15:39:09.8\tlog_raw\tgps_raw\t#INSPVAXA,USB3,0,48.0,FINESTEERING,2107,283167.800,02000000,471d,15824;INS_ALIGNMENT_COMPLETE,INS_RTKFIXED,37.37108803292,126.72336912346,8.2209,22.3000,0.0149,0.0089,-0.0014,-0.377171042,-0.586737055,287.872482646,0.2105,0.1573,0.2615,0.0344,0.0343,0.0312,0.0793,0.0803,5.0087,0f000005,0*c60ea973\n\tsystem status\tnormal 2 28.000000 0 0\trobot status\t224.459196\t106.302079\t8.220900\t-0.377171\t-0.586737\t162.127517\t0.000000\t0.000000\n\t\n15:39:10.3\tlog_raw\tgps_raw\t#INSPVAXA,USB3,0,42.0,FINESTEERING,2107,283168.300,02000000,471d,15824;INS_ALIGNMENT_COMPLETE,INS_RTKFIXED,37.37108803880,126.72336912583,8.2209,22.3000,0.0161,0.0086,-0.0017,-0.375595415,-0.586259403,287.874300642,0.2244,0.1729,0.2724,0.0385,0.0383,0.0343,0.0796,0.0805,5.0113,0f000005,0*8044c93c\n\tsystem status\tnormal 2 28.000000 0 0\trobot status\t224.459406\t106.302732\t8.220900\t-0.375595\t-0.586259\t162.125699\t0.000000\t0.000000\n\t\n15:39:10.8\tlog_raw\tgps_raw\t#INSPVAXA,USB3,0,42.0,FINESTEERING,2107,283168.800,02000000,471d,15824;INS_ALIGNMENT_COMPLETE,INS_RTKFIXED,37.37108800795,126.72336909694,8.2215,22.3000,0.0141,0.0074,-0.0014,-0.380382564,-0.586190595,287.878476093,0.2244,0.1729,0.2724,0.0385,0.0383,0.0343,0.0796,0.0805,5.0113,0f000005,0*54eab961\n\tsystem status\tnormal 2 28.000000 0 0\trobot status\t224.456847\t106.299308\t8.221500\t-0.380383\t-0.586191\t162.121524\t0.000000\t0.000000\n\t\n15:39:11.3\tlog_raw\tgps_raw\t#INSPVAXA,USB3,0,47.5,FINESTEERING,2107,
